vi "osd_send_data.vi"(4 "COM":bool, 5 "bypara":u8, 6 "VISA name":refnum<visa-resource-name>, 7 "byIndex":u8, 9 "pbyData":u8[](array[numeric]), 10 "bySubcmd":u8, 11 "byCmd":u8) -> (3 "return":i32)   [LabVIEW 2016]
panel:
  in  "vdcmd_info_osd_t":T1
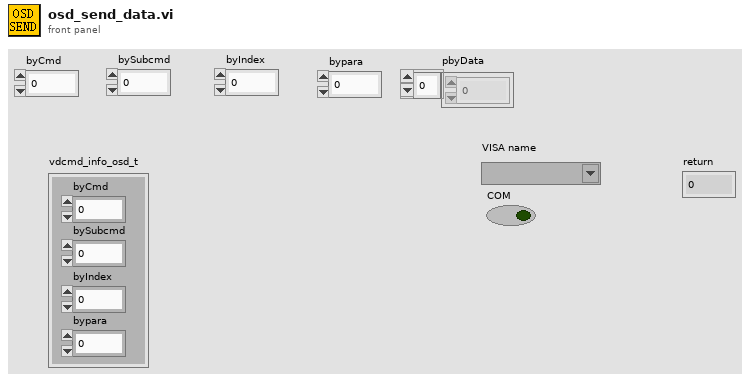
[diagram p1: front panel]
types:
  T1 = cluster{"byCmd":u8, "bySubcmd":u8, "byIndex":u8, "bypara":u8}
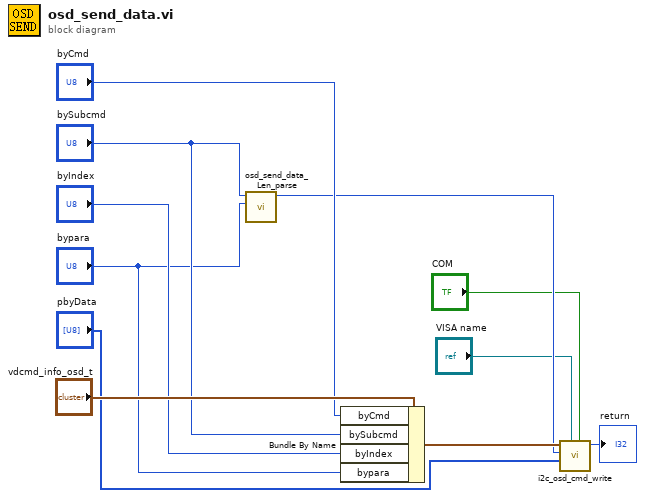
[diagram p0: block diagram]
diagram:
  n1 = call "osd_send_data_Len_parse.vi"("bypara"="bypara", "bySubcmd"="bySubcmd") -> ("byDataLen"=w5:u8)  [unwired: 9 in]
  n2 = Bundle By Name(cluster="vdcmd_info_osd_t", "byCmd"="byCmd", "bySubcmd"="bySubcmd", "byIndex"="byIndex", "bypara"="bypara") -> (w6:T1)
  n3 = call "i2c_osd_cmd_write.vi"("COM"="COM", "VISA name"="VISA name", "data"="pbyData", "byDataLen"=w5, "vdcmd_info_osd_t"=w6) -> ("return"=→"return":i32)  [unwired: 6 in]
